vi "Get Send Message Queue.vi"(8 "error in":errorcluster) -> (0 "error out":errorcluster, 3 "send queue":refnum<queue>)   [LabVIEW 2016, in "Vision Server.lvclass"]
uses:
  Vision Server.lvclass
  typedef/Message Type.ctl
  Vision Server.lvclass/Vision Server.ctl
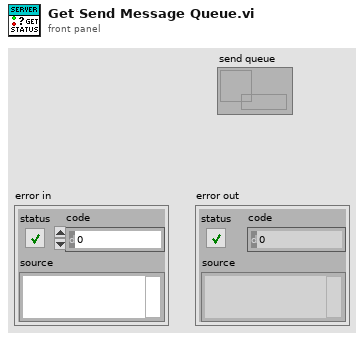
[diagram p1: front panel]
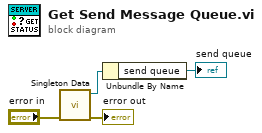
[diagram p0: block diagram]
diagram:
  n1 = call "Singleton Data.vi"("error in"="error in") -> ("error out"=→"error out":errorcluster, "Vision Server Copy"=w4:refnum<class "Vision Server.lvclass">)  [unwired: 9 in]
  n2 = Unbundle By Name(w4) -> ("send queue"=→"send queue":refnum<queue>)
